vi "Parse Cargo Bay Digital Inputs.vi"(11 "stream in":u8[](array[numeric])) -> (0 "Cargo Bay Digital Inputs":T1, 3 "stream out":u8[](array[numeric]))   [LabVIEW 2014]
doc: "Read the state of the cargo bay digital inputs from a UART data stream."
uses:
  Cargo Bay Digital Inputs.ctl
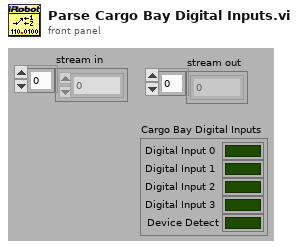
[diagram p1: front panel]
types:
  T1 = typedef "Cargo Bay Digital Inputs.ctl" = cluster{"Digital Input 0":bool, "Digital Input 1":bool, "Digital Input 2":bool, "Digital Input 3":bool, "Device Detect":bool}
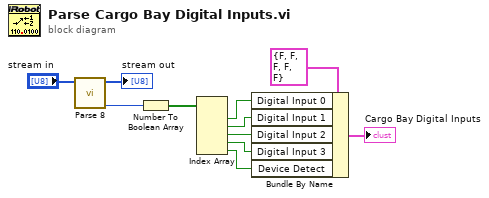
[diagram p0: block diagram]
diagram:
  n1 = call "Parse 8.vi"("stream in"="stream in") -> ("value"=w1:u8, "stream out"=→"stream out":u8[])  [unwired: 9 out]
  n2 = Number To Boolean Array(number=w1) -> (Boolean array=w11:bool[])
  n3 = Index Array(array=w11) -> (element #1=w10:bool, element #2=w9:bool, element #3=w8:bool, element #4=w7:bool, element #5=w6:bool)  [unwired: 5 in]
  n4 = Bundle By Name(cluster=T1 {"Digital Input 0"=FALSE, "Digital Input 1"=FALSE, "Digital Input 2"=FALSE, "Digital Input 3"=FALSE, "Device Detect"=FALSE} ("Cargo Bay Digital Inputs"), "Digital Input 0"=w10, "Digital Input 1"=w9, "Digital Input 2"=w8, "Digital Input 3"=w7, "Device Detect"=w6) -> (→"Cargo Bay Digital Inputs":T1)
